vi "LS340_ReadSensor.vi"(0 "VISA resource name":refnum<visa-resource-name>, 7 "Input (0: A)":u16(ring) items=["A", "B", "C", "D"], 11 "error in (no error)":errorcluster) -> (4 "VISA resource name out":refnum<visa-resource-name>, 6 "Celsius Reading":dbl min=-273.16 max=1372.0 step=1e-05 format="%^.5e", 8 "Kelvin Reading":dbl min=0.0 max=1645.0 step=1e-05 format="%^.5e", 10 "Sensor Units Reading":dbl min=-7.5 max=300000.0 step=1e-05 format="%^.5e", 15 "error out":errorcluster)   [LabVIEW 2012]
doc: "This VI querys the instrument for an inputs sensor reading in Celsius, Kelvin, and Sensor Units."
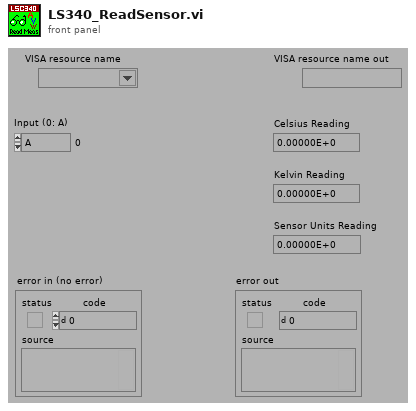
[diagram p1: front panel]
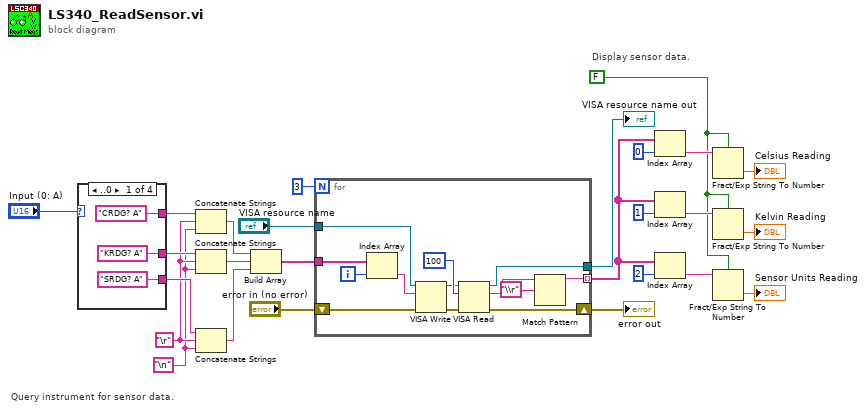
[diagram p0: block diagram]
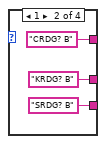
[diagram p2: hidden frame]
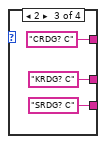
[diagram p3: hidden frame]
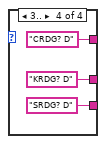
[diagram p4: hidden frame]
diagram:
  w1 = "\n"
  w2 = "\r"
  w9 = FALSE ("use system decimal point (T)")
  # "Query instrument for sensor data."
  # "Display sensor data."
  n1 = case shown="..0" "Input (0: A)" {
    tunnel: ["CRDG? A" "CRDG? B" "CRDG? C" "CRDG? D"] -> w8
    tunnel: ["KRDG? A" "KRDG? B" "KRDG? C" "KRDG? D"] -> w7
    tunnel: ["SRDG? A" "SRDG? B" "SRDG? C" "SRDG? D"] -> w6
    frame ..0 {
    }
    frame 1 {
    }
    frame 2 {
    }
    frame 3.. {
    }
  }
  n2 = Concatenate Strings(w8, w2, w1) -> (w5:string)
  n3 = Concatenate Strings(w7, w2, w1) -> (w4:string)
  n4 = Concatenate Strings(w6, w2, w1) -> (w3:string)
  n5 = Build Array(w5, w4, w3) -> (w16:string[])
  n6 = for {
    N: 3 -> [_]
    tunnel: w16 -> [w48]
    shift-right: [w45] -> w12
    shift-left: "error in (no error)" -> [w46]
    tunnel: [w44] -> w11
    tunnel: "VISA resource name" -> [w43]
    tunnel: [w41] -> w10 mode=indexing
    i -> [w47]
    n7 = Index Array(array=w48, index=w47) -> (element=w39:string)
    n8 = VISA Write(VISA resource name=w43, write buffer=w39, error in (no error)=w46) -> (VISA resource name out=w40:refnum<visa-resource-name>, error out=w51:errorcluster)  [unwired: 1 out]
    n9 = VISA Read(VISA resource name=w40, byte count=100, error in (no error)=w51) -> (VISA resource name out=w44:refnum<visa-resource-name>, read buffer=w49:string, error out=w45:errorcluster)  [unwired: 1 out]
    n10 = Match Pattern(string=w49, regular expression="\\r") -> (before substring=w41:string)  [unwired: 1 in, 3 out]
  }
  "VISA resource name out" <- w11
  "error out" <- w12
  n11 = Index Array(array=w10, index=0) -> (element=w21:string)
  n12 = Index Array(array=w10, index=1) -> (element=w22:string)
  n13 = Index Array(array=w10, index=2) -> (element=w23:string)
  n14 = Fract/Exp String To Number(use system decimal point (T)=w9, string=w21) -> (number=→"Celsius Reading":dbl)  [unwired: 2 in, 1 out]
  n15 = Fract/Exp String To Number(use system decimal point (T)=w9, string=w22) -> (number=→"Kelvin Reading":dbl)  [unwired: 2 in, 1 out]
  n16 = Fract/Exp String To Number(use system decimal point (T)=w9, string=w23) -> (number=→"Sensor Units Reading":dbl)  [unwired: 2 in, 1 out]
